vi "pp2_wrapMsTimes.vi"(4 "Exit cum ms":i64, 6 "Cum ms":i64, 7 "Curr ms":i64) -> (0 "Exit?":bool, 1 "Run loop diff":i64, 2 "Cum ms (updated)":i64, 3 "Curr ms (updated)":i64)   [LabVIEW 2013]
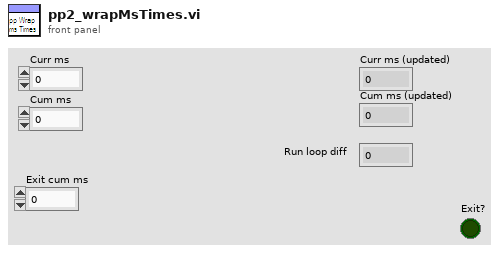
[diagram p1: front panel]
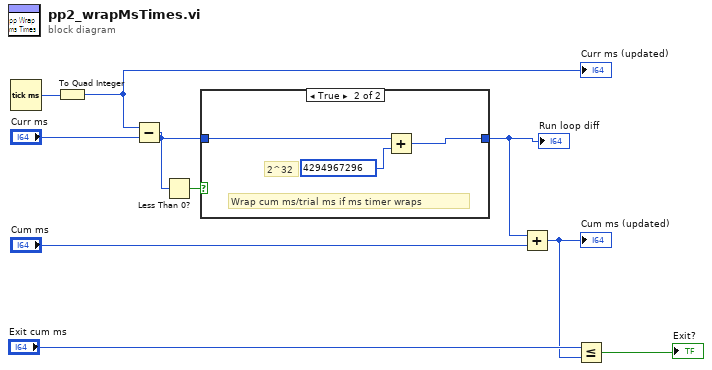
[diagram p0: block diagram]
diagram:
  n1 = Tick Count (ms)() -> (millisecond timer value=w10:u32)
  n2 = To Quad Integer(1:w10) -> (0:w6:i64)
  "Curr ms (updated)" <- w6
  n3 = Subtract(x=w6, y="Curr ms") -> (x-y=w3:i64)
  n4 = Less Than 0?(x=w3) -> (x < 0?=w4:bool)
  n5 = case shown="True" w4 {
    tunnel: w3 -> [w11 w13]
    tunnel: [w11 w14] -> w1
    frame False {
    }
    frame True {
      # "Wrap cum ms/trial ms if ms timer wraps"
      # "2^32"
      n6 = Add(x=w13, y=i64 4294967296) -> (x+y=w14:i64)
    }
  }
  "Run loop diff" <- w1
  n7 = Add(x=w1, y="Cum ms") -> (x+y=w2:i64)
  "Cum ms (updated)" <- w2
  n8 = Less Or Equal?(x="Exit cum ms", y=w2) -> (x <= y?=→"Exit?":bool)
